vi "LeapMotion.vi"(8 "Error In":errorcluster) -> (0 "Error Out":errorcluster, 2 "x-y 2":cluster{"X":sgl, "Y":sgl, "Z":sgl})   [LabVIEW 2014]
uses:
  <vilib>/MakerHub/Leap/Public/Instance VIs/Read 1 Hand Position Velocity.vi
  <vilib>/MakerHub/Leap/Public/Gestures/Key Tap/Instance VIs/Read 1 Key Tap Position.vi
  libraryGcode/variableGlobal/StartAutoandGcode.vi
  libraryGcode/LibraryGcode.lvlib
  <vilib>/MakerHub/Leap/Private/Type Defs/Gesture State.ctl
panel:
  out "Key Tap Status":T1
  out "x-y":cluster{"X":sgl, "Y":sgl, "Z":sgl}
  in  "Hand Position OLD":cluster{"X":sgl, "Y":sgl, "Z":sgl}
  out "Enum":T2(ring)
  out "Hand Position":cluster{"X":sgl, "Y":sgl, "Z":sgl}
  in  "stop":bool
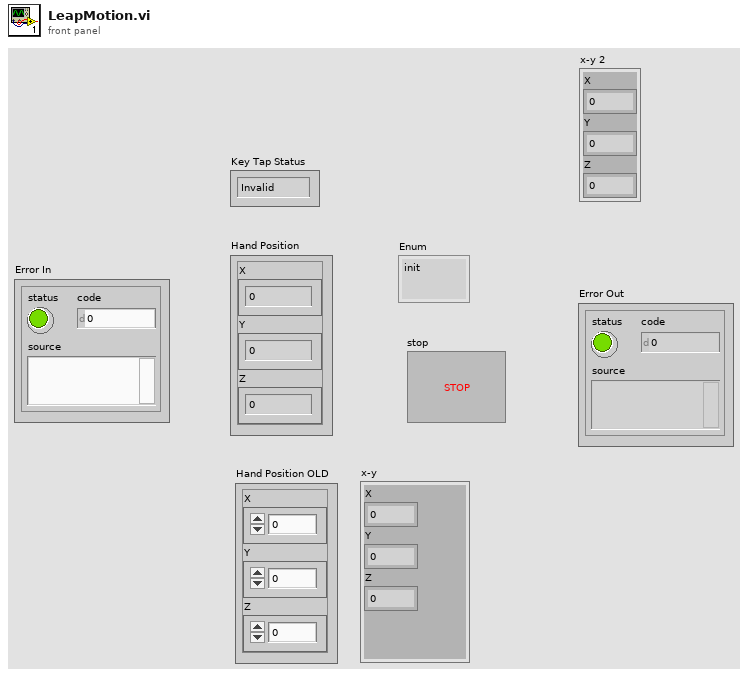
[diagram p1: front panel]
types:
  T1 = typedef "LMH-Leap.lvlib/Gesture State.ctl" = enum16{"Invalid", "Start", "Update", "Stop"}
  T2 = enum16{"init", "Wait", "GetdataHand", "CompareData", "Move", "Finish"}
  T3 = typedef "LMH-Leap.lvlib/Leap Handle.ctl" = cluster{"LeapCSharp":refnum<k24>}
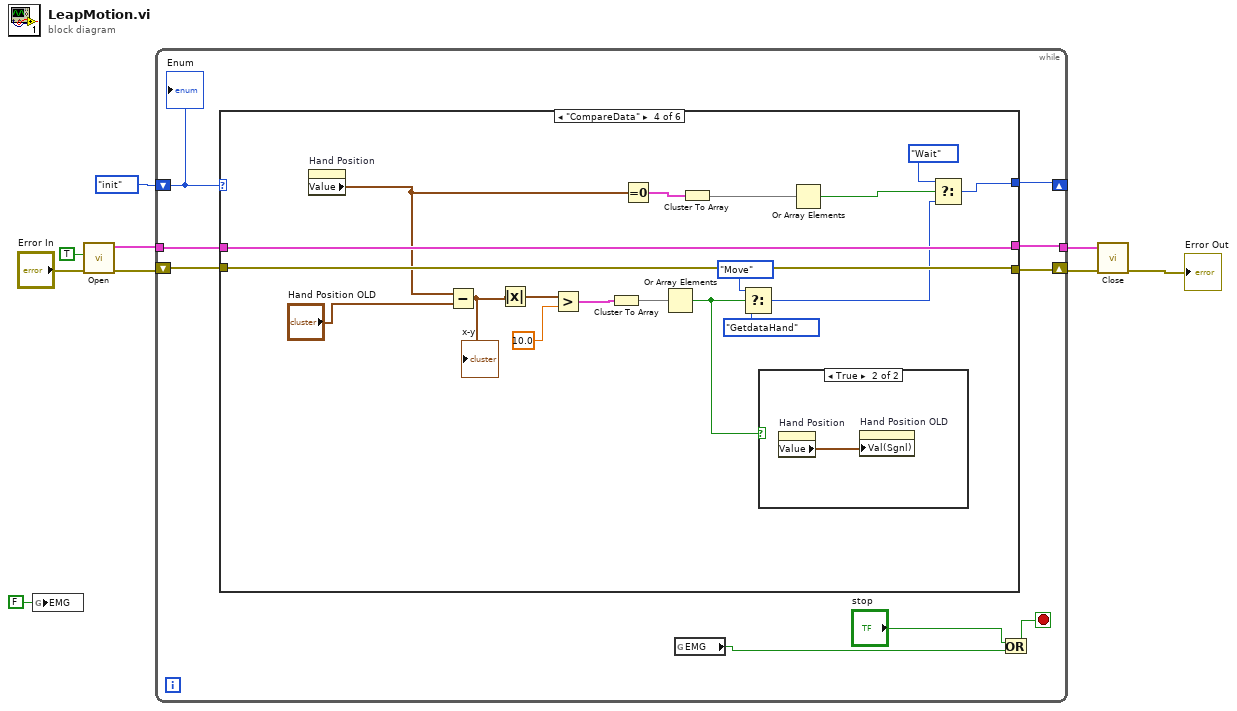
[diagram p0: block diagram]
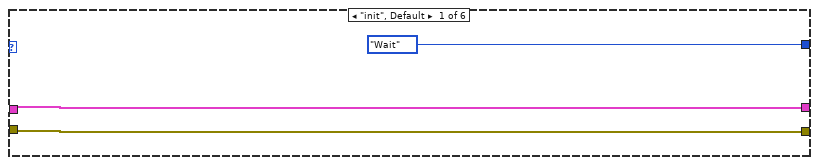
[diagram p2: hidden frame]
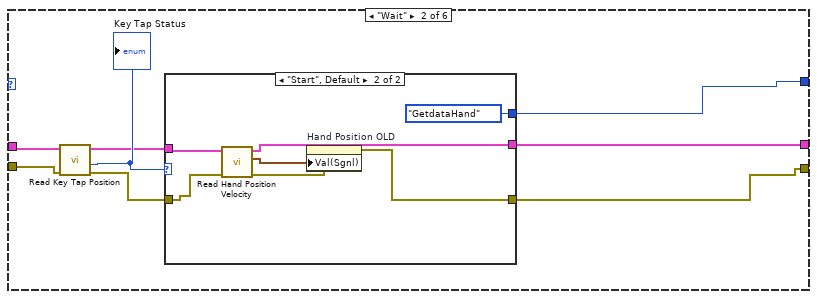
[diagram p3: hidden frame]
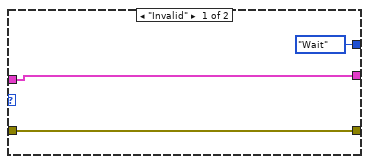
[diagram p4: hidden frame]
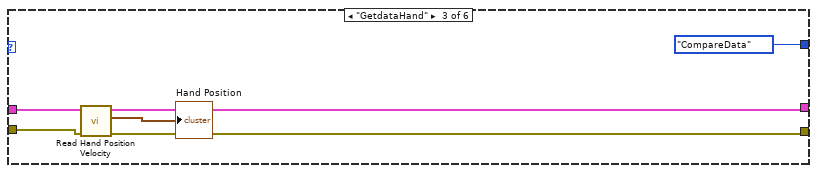
[diagram p5: hidden frame]
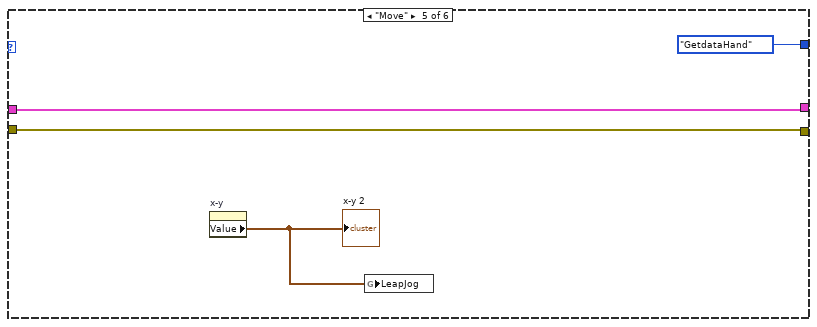
[diagram p7: hidden frame]
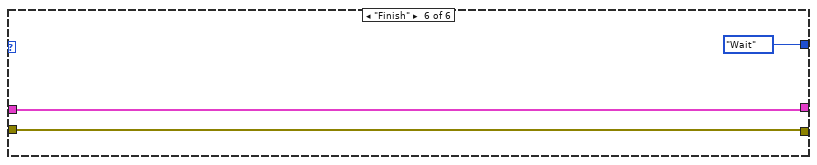
[diagram p8: hidden frame]
diagram:
  n1 = global write "StartAutoandGcode.vi" "EMG"(FALSE ("EMG")) -> ()
  n2 = call <vilib>:"Open.vi"("Error In"="Error In", "Enable Gestures? (T)"=TRUE) -> ("Error Out"=w5:errorcluster, "Leap Handle"=w6:T3)  [unwired: 8 in]
  n3 = while {
    shift-right: [w13] -> _
    shift-left: T2."init" -> [w14]
    shift-right: [w16] -> w7
    shift-left: w5 -> [w18]
    tunnel: w6 -> [w17]
    tunnel: [w15] -> w8
    stop <- w11 stop-if-true
    n4 = case shown="\"CompareData\"" w14 {
      tunnel: w18 -> [w19 w28 w44 w58 w67 w70]
      tunnel: w17 -> [w20 w29 w45 w59 w68 w71]
      tunnel: [w19 w23 w42 w58 w67 w70] -> w16
      tunnel: [w20 w24 w43 w59 w68 w71] -> w15
      tunnel: [T2."Wait" w26 T2."CompareData" w60 T2."GetdataHand" T2."Wait"] -> w13
      frame "init", Default {
      }
      frame "Wait" {
        n5 = call-poly <vilib>:"Read Key Tap Position.vi"("Error In"=w28, "Leap Handle"=w29) -> ("Error Out"=w22:errorcluster, "Key Tap Status"=w27:T1, "Leap Handle"=w25:T3)  [unwired: 6 in, 1 out]
        "Key Tap Status" <- w27
        n6 = case shown="\"Start\", Default" w27 {
          tunnel: [T2."Wait" T2."GetdataHand"] -> w26
          tunnel: w25 -> [w31 w38]
          tunnel: [w31 w37] -> w24
          tunnel: [w30 w33] -> w23
          tunnel: w22 -> [w30 w36]
          frame "Invalid" {
          }
          frame "Start", Default {
            n7 = call-poly <vilib>:"Read Hand Position Velocity.vi"("Error In"=w36, "Leap Handle"=w38) -> ("Error Out"=w34:errorcluster, "Hand Position"=w35:cluster{"X":sgl, "Y":sgl, "Z":sgl}, "Leap Handle"=w37:T3)  [unwired: 6 in, 1 out]
            n8 = property on="Hand Position OLD" class="Clust (strict)"(error in=w34, "Val(Sgnl)"=w35) -> (error out=w33:errorcluster)  [unwired: 1 in, 1 out]
          }
        }
      }
      frame "GetdataHand" {
        n9 = call-poly <vilib>:"Read Hand Position Velocity.vi"("Error In"=w44, "Leap Handle"=w45) -> ("Error Out"=w42:errorcluster, "Hand Position"=→"Hand Position":cluster{"X":sgl, "Y":sgl, "Z":sgl}, "Leap Handle"=w43:T3)  [unwired: 6 in, 1 out]
      }
      frame "CompareData" {
        n10 = property on="Hand Position" class="Clust (strict)"() -> ("Value"=w57:cluster{"X":sgl, "Y":sgl, "Z":sgl})  [unwired: 2 in, 2 out]
        n11 = Subtract(x=w57, y="Hand Position OLD") -> (x-y=w47:cluster{"X":sgl, "Y":sgl, "Z":sgl})
        "x-y" <- w47
        n12 = Absolute Value(x=w47) -> (abs(x)=w46:cluster{"X":sgl, "Y":sgl, "Z":sgl})
        n13 = Greater?(x=w46, y=10.0) -> (0:w54:cluster{"X":bool, "Y":bool, "Z":bool})
        n14 = Cluster To Array(cluster=w54) -> (array=w53:bool[])
        n15 = Equal To 0?(x=w57) -> (x = 0?=w63:cluster{"X":bool, "Y":bool, "Z":bool})
        n16 = Or Array Elements(Boolean array=w53) -> (logical OR=w48:bool)
        n17 = Cluster To Array(cluster=w63) -> (array=w49:bool[])
        n18 = Select(t=T2."Move", s=w48, f=T2."GetdataHand") -> (s? t:f=w50:T2)
        n19 = case shown="True" w48 {
          frame False {
          }
          frame True {
            n20 = property on="Hand Position" class="Clust (strict)"() -> ("Value"=w64:cluster{"X":sgl, "Y":sgl, "Z":sgl})  [unwired: 2 in, 2 out]
            n21 = property on="Hand Position OLD" class="Clust (strict)"("Val(Sgnl)"=w64) -> ()  [unwired: 2 in, 2 out]
          }
        }
        n22 = Or Array Elements(Boolean array=w49) -> (logical OR=w62:bool)
        n23 = Select(t=T2."Wait", s=w62, f=w50) -> (s? t:f=w60:T2)
      }
      frame "Move" {
        n24 = property on="x-y" class="Clust (strict)"() -> ("Value"=w65:cluster{"X":sgl, "Y":sgl, "Z":sgl})  [unwired: 2 in, 2 out]
        "x-y 2" <- w65
        n25 = global write "StartAutoandGcode.vi" "LeapJog"(w65) -> ()
      }
      frame "Finish" {
      }
    }
    n26 = global read "StartAutoandGcode.vi" "EMG"() -> (w10:bool)
    n27 = Or(x="stop", y=w10) -> (x .or. y?=w11:bool)
    "Enum" <- w14
  }
  n28 = call <vilib>:"Close.vi"("Error In"=w7, "Leap Handle"=w8) -> ("Error Out"=→"Error Out":errorcluster)  [unwired: 9 in]
